vi "2 Singles Make Double.vi"(9 "Value":T1, 10 "Reverse In":T2={"DevStatus"={"status"=FALSE, "code"=0, "source"=""}, "Pneumatics Control Module"=0, "Forward Solenoid Channel"=enum."Invalid", "Reverse Solenoid Channel"=enum."Invalid"}, 11 "Forward In":T2={"DevStatus"={"status"=FALSE, "code"=0, "source"=""}, "Pneumatics Control Module"=0, "Forward Solenoid Channel"=enum."Invalid", "Reverse Solenoid Channel"=enum."Invalid"}) -> (2 "Reverse Out":T2={"DevStatus"={"status"=FALSE, "code"=0, "source"=""}, "Pneumatics Control Module"=0, "Forward Solenoid Channel"=enum."Invalid", "Reverse Solenoid Channel"=enum."Invalid"}, 3 "Forward Out":T2={"DevStatus"={"status"=FALSE, "code"=0, "source"=""}, "Pneumatics Control Module"=0, "Forward Solenoid Channel"=enum."Invalid", "Reverse Solenoid Channel"=enum."Invalid"})   [LabVIEW 2014]
uses:
  <vilib>/Rock Robotics/WPI/Solenoid/WPI_SolenoidValue.ctl
  <vilib>/Rock Robotics/WPI/Solenoid/WPI_SolenoidDevRef.ctl
  <vilib>/Rock Robotics/WPI/Solenoid/WPI_SolenoidChannel.ctl
  <vilib>/Rock Robotics/WPI/Solenoid/WPI_SolenoidSetEnum.vi
panel:
  out "Forward State":T1
  out "Reverse State":T1
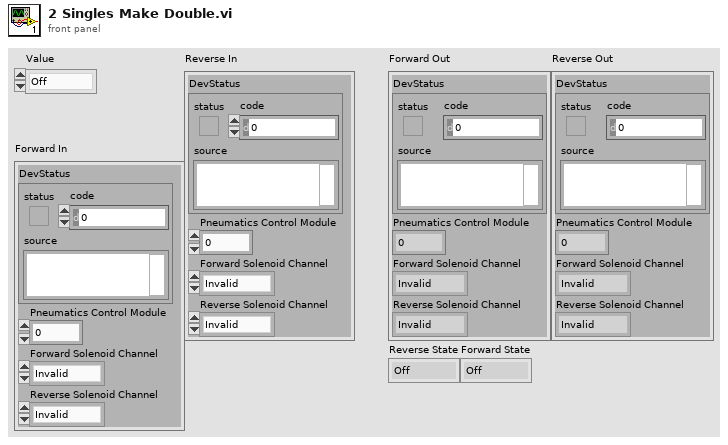
[diagram p1: front panel]
types:
  T1 = typedef "WPI_SolenoidValue.ctl" = enum16{"Off", "On", "Forward", "Reverse"}
  T2 = typedef "WPI_SolenoidDevRef.ctl" = cluster{"DevStatus":errorcluster, "Pneumatics Control Module":u8, "Forward Solenoid Channel":T3, "Reverse Solenoid Channel":T3}
  T3 = typedef "WPI_SolenoidChannel.ctl" = enum8{"Solenoid 0", "Solenoid 1", "Solenoid 2", "Solenoid 3", "Solenoid 4", "Solenoid 5", "Solenoid 6", "Solenoid 7", "Invalid"}
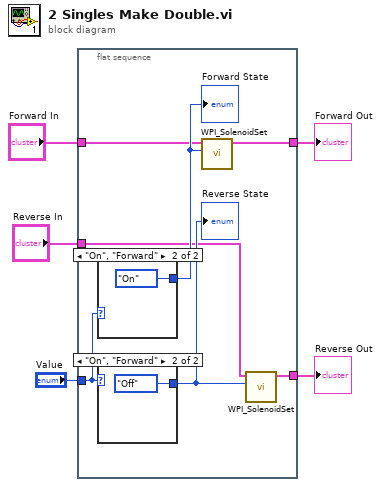
[diagram p0: block diagram]
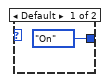
[diagram p2: hidden frame]
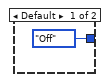
[diagram p3: hidden frame]
diagram:
  n1 = flat-sequence {
    tunnel: "Forward In" -> [w7]
    tunnel: "Reverse In" -> [w6]
    tunnel: "Value" -> [w12]
    tunnel: [w11] -> w4
    tunnel: [w10] -> w3
    frame #0 {
      n2 = case shown="\"On\", \"Forward\"" w12 {
        tunnel: [WPI_SolenoidValue."Off" ("Value 2") WPI_SolenoidValue."On" ("Value 2")] -> w9
        frame Default {
        }
        frame "On", "Forward" {
        }
      }
      "Forward State" <- w9
      n3 = case shown="\"On\", \"Forward\"" w12 {
        tunnel: [WPI_SolenoidValue."On" ("Value 2") WPI_SolenoidValue."Off" ("Value 2")] -> w8
        frame Default {
        }
        frame "On", "Forward" {
        }
      }
      "Reverse State" <- w8
      n4 = call-poly <vilib>:"WPI_SolenoidSet.vi"("Value"=w9, "SolenoidDevRef"=w7) -> ("SolenoidDevRef"=w11:T2)  [unwired: 8 in, 1 out]
      n5 = call-poly <vilib>:"WPI_SolenoidSet.vi"("Value"=w8, "SolenoidDevRef"=w6) -> ("SolenoidDevRef"=w10:T2)  [unwired: 8 in, 1 out]
    }
  }
  "Forward Out" <- w4
  "Reverse Out" <- w3
